vi "ReadWrite Top Level.vi"(5 "Late?":bool, 6 "Iteration":i32, 7 "Mode":T16, 8 "error in (no error)":errorcluster, 9 "Iteration Duration":i64, 11 "RT Data in":T1 {"Label Transfer Config"."Block Data Refs"."Data Reference" format="%.0x"; "Status Config"."HWOut Dur Ref" format="%.0x"; "Status Config"."HWIn Dur Ref" format="%.0x"; "Status Config"."HWOut Count Ref" format="%.0x"; "Status Config"."HWIn Count Ref" format="%.0x"; "Status Config"."Error Data Ref" format="%.0x"; "HWOutput Channels"."Labels Settings"."Driver Data"."Num Bits" min=1 max=32; "HWOutput Channels"."Labels Settings"."Driver Data"."Start Bit" min=8 max=31; "HWOutput Channels"."Labels Settings"."Block Data Refs"."Data Reference" format="%.0x"; "HWOutput Channels"."Labels Settings"."Label" format="%.0o"; "HWInput Channels"."Labels Settings"."Driver Data"."Num Bits" min=1 max=32; "HWInput Channels"."Labels Settings"."Driver Data"."Start Bit" min=8 max=31; "HWInput Channels"."Labels Settings"."Block Data Refs"."Data Reference" format="%.0x"; "HWInput Channels"."Labels Settings"."Label" format="%.0o"}) -> (0 "error out":errorcluster, 3 "RT Data out":T1 {"Label Transfer Config"."Block Data Refs"."Data Reference" format="%.0x"; "Status Config"."HWOut Dur Ref" format="%.0x"; "Status Config"."HWIn Dur Ref" format="%.0x"; "Status Config"."HWOut Count Ref" format="%.0x"; "Status Config"."HWIn Count Ref" format="%.0x"; "Status Config"."Error Data Ref" format="%.0x"; "HWOutput Channels"."Labels Settings"."Driver Data"."Num Bits" min=1 max=32; "HWOutput Channels"."Labels Settings"."Driver Data"."Start Bit" min=8 max=31; "HWOutput Channels"."Labels Settings"."Block Data Refs"."Data Reference" format="%.0x"; "HWOutput Channels"."Labels Settings"."Label" format="%.0o"; "HWInput Channels"."Labels Settings"."Driver Data"."Num Bits" min=1 max=32; "HWInput Channels"."Labels Settings"."Driver Data"."Start Bit" min=8 max=31; "HWInput Channels"."Labels Settings"."Block Data Refs"."Data Reference" format="%.0x"; "HWInput Channels"."Labels Settings"."Label" format="%.0o"})   [LabVIEW 2011, in "AIT 1553 Custom Device.lvlib"]
uses:
  AIT 1553 Custom Device.lvlib
  RT Controls/ReadWrite Selector.ctl
  RT Controls/RT Data.ctl
  RT Controls/RT HW Channel.ctl
  RT Controls/RT Label Settings.ctl
  Controls and Global/Label.ctl
  Controls and Global/transferPeriod.ctl
  <vilib>/NI Veristand/Custom Device API/Block Data Reference.ctl
  <vilib>/NI Veristand/Custom Device API/Data Reference.ctl
  RT Controls/Driver Data.ctl
  Controls and Global/Start Bit.ctl
  Controls and Global/Number of Bits.ctl
  RT Controls/Error Qs.ctl
  RT Controls/Status Channels Config.ctl
  RT Controls/FIFO.ctl
  RT Controls/Label Transfer Config.ctl
  <userlib>/ARINC-429/vi/enum/Owl429HardwareSource.ctl
  <vilib>/NI Veristand/Custom Device API/NI VeriStand - Set Channel Value by Data Reference.vi
  <vilib>/NI Veristand/Custom Device API/NI VeriStand - Get Channel Values by Block Data Reference.vi
  <vilib>/NI Veristand/Custom Device API/Global Data Refs.vi
  <vilib>/NI Veristand/Custom Device API/Custom Device API.lvlib
  <userlib>/ARINC-429/Owl429.lvlib
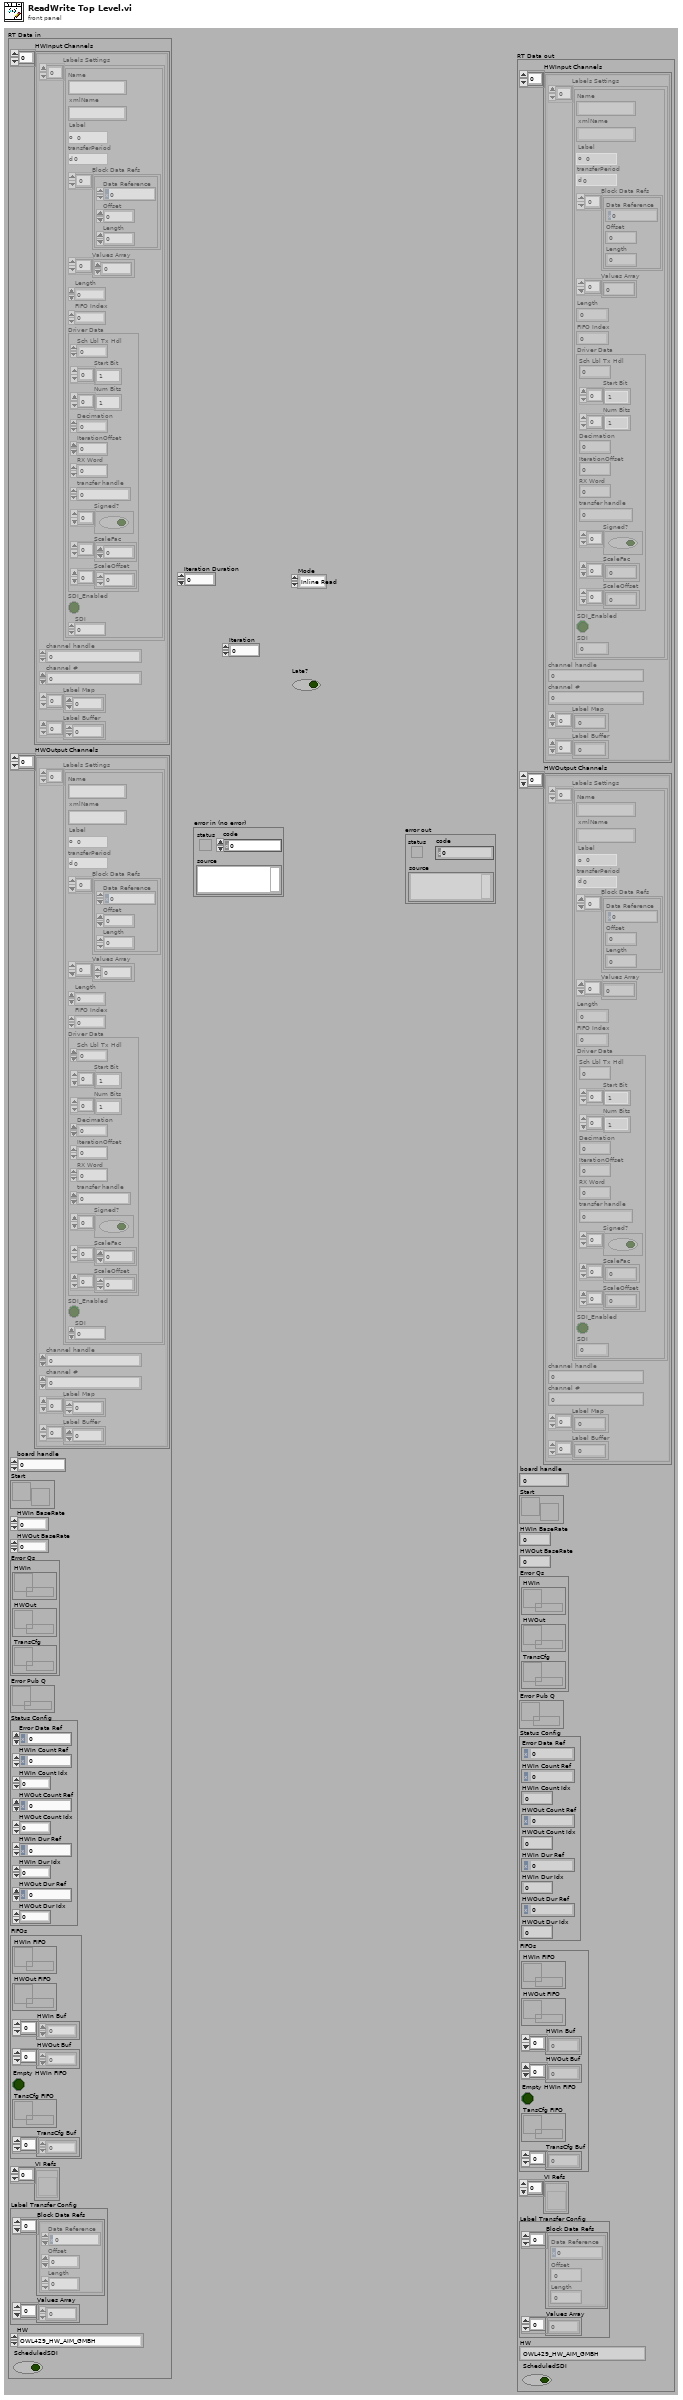
[diagram p1: front panel]
types:
  T1 = typedef "AIT 1553 Custom Device.lvlib/RT Data.ctl" = cluster{"HWInput Channels":T2[], "HWOutput Channels":T2[], "board handle":u32, "Start":refnum<notifier>, "HWIn BaseRate":i64, "HWOut BaseRate":i64, "Error Qs":T11, "Error Pub Q":refnum<queue>, "Status Config":T12, "FIFOs":T13, "VI Refs":refnum<vi>[], "Label Transfer Config":T14, "HW":T15, "ScheduledSDI":bool}
  T2 = typedef "AIT 1553 Custom Device.lvlib/RT HW Channel.ctl" = cluster{"Labels Settings":T3[], "channel handle":u32, "channel #":u16, "Label Map":i32[], "Label Buffer":u32[]}
  T3 = typedef "AIT 1553 Custom Device.lvlib/RT Label Settings.ctl" = cluster{"Name":string, "xmlName":string, "Label":T4, "transferPeriod":T5, "Block Data Refs":T6[], "Values Array":dbl[], "Length":i32, "FIFO Index":i32, "Driver Data":T8, "SDI_Enabled":bool, "SDI":u8}
  T4 = typedef "AIT 1553 Custom Device.lvlib/Label.ctl" = u8
  T5 = typedef "AIT 1553 Custom Device.lvlib/transferPeriod.ctl" = u32
  T6 = typedef "Custom Device API.lvlib/Block Data Reference.ctl" = cluster{"Data Reference":T7, "Offset":i32, "Length":i32}
  T7 = typedef "Custom Device API.lvlib/Data Reference.ctl" = i32
  T8 = typedef "AIT 1553 Custom Device.lvlib/Driver Data.ctl" = cluster{"Sch Lbl Tx Hdl":u32, "Start Bit":T9[], "Num Bits":T10[], "Decimation":i32, "IterationOffset":i32, "RX Word":u32, "transfer handle":u32, "Signed?":bool[], "ScaleFac":dbl[], "ScaleOffset":dbl[]}
  T9 = typedef "AIT 1553 Custom Device.lvlib/Start Bit.ctl" = i32
  T10 = typedef "AIT 1553 Custom Device.lvlib/Number of Bits.ctl" = i32
  T11 = typedef "AIT 1553 Custom Device.lvlib/Error Qs.ctl" = cluster{"HWIn":refnum<queue>, "HWOut":refnum<queue>, "TransCfg":refnum<queue>}
  T12 = typedef "AIT 1553 Custom Device.lvlib/Status Channels Config.ctl" = cluster{"Error Data Ref":T7, "HWIn Count Ref":T7, "HWIn Count Idx":i32, "HWOut Count Ref":T7, "HWOut Count Idx":i32, "HWIn Dur Ref":T7, "HWIn Dur Idx":i32, "HWOut Dur Ref":T7, "HWOut Dur Idx":i32}
  T13 = typedef "AIT 1553 Custom Device.lvlib/FIFO.ctl" = cluster{"HWIn FIFO":refnum<k33>, "HWOut FIFO":refnum<k33>, "HWIn Buf":dbl[], "HWOut Buf":dbl[], "Empty HWIn FIFO":bool, "TansCfg FIFO":refnum<k33>, "TransCfg Buf":dbl[]}
  T14 = typedef "AIT 1553 Custom Device.lvlib/Label Transfer Config.ctl" = cluster{"Block Data Refs":T6[], "Values Array":dbl[]}
  T15 = typedef "Owl429.lvlib/Owl429HardwareSource.ctl" = enum16{"OWL429_HW_AIM_GMBH", "OWL429_HW_AIT"}
  T16 = typedef "AIT 1553 Custom Device.lvlib/ReadWrite Selector.ctl" = enum16{"Inline Read", "Inline Write", "Async HWIn", "Async HWOut"}
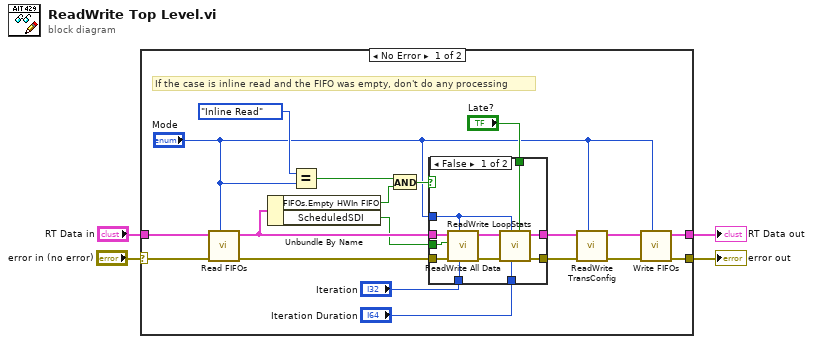
[diagram p0: block diagram]
diagram:
  n1 = case shown="No Error" "error in (no error)" {
    selector: "error in (no error)" -> [w13 w38]
    tunnel: "RT Data in" -> [w23 w37]
    tunnel: [w22 w37] -> w3
    tunnel: [w21 w38] -> w2
    frame No Error {
      # "If the case is inline read and the FIFO was empty, don't do any processing"
      n2 = call "Read FIFOs.vi"("Mode"="Mode", "error in (no error)"=w13, "RT Data in"=w23) -> ("error out"=w20:errorcluster, "RT Data out"=w17:T1)  [unwired: 7 in]
      n3 = Unbundle By Name(w17) -> ("FIFOs.Empty HWIn FIFO"=w16:bool, "ScheduledSDI"=w5:bool)
      n4 = Equal?(x=ReadWrite_Selector."Inline Read", y="Mode") -> (x = y?=w18:bool)
      n5 = And(x=w18, y=w16) -> (x .and. y?=w15:bool)
      n6 = case shown="False" w15 {
        tunnel: w20 -> [w34 w36]
        tunnel: [w29 w36] -> w10
        tunnel: [w28 w35] -> w9
        tunnel: w17 -> [w33 w35]
        tunnel: "Mode" -> [w26 _]
        tunnel: "Iteration" -> [w32 _]
        tunnel: "Late?" -> [w27 _]
        tunnel: "Iteration Duration" -> [w25 _]
        tunnel: w5 -> [w24 _]
        frame False {
          n7 = call "ReadWrite All Data.vi"("Iteration"=w32, "Mode"=w26, "error in (no error)"=w34, "ScheduledSDI"=w24, "RT Data in"=w33) -> ("error out"=w30:errorcluster, "RT Data out"=w31:T1)  [unwired: 5 in]
          n8 = call "ReadWrite LoopStats.vi"("Late"=w27, "Iteration Duration"=w25, "Mode"=w26, "error in (no error)"=w30, "RT Data in"=w31) -> ("error out"=w29:errorcluster, "RT Data out"=w28:T1)  [unwired: 5 in]
        }
        frame True {
        }
      }
      n9 = call "ReadWrite TransConfig.vi"("Mode"="Mode", "error in (no error)"=w10, "RT Data in"=w9) -> ("error out"=w6:errorcluster, "RT Data out"=w7:T1)  [unwired: 7 in]
      n10 = call "Write FIFOs.vi"("Mode"="Mode", "error in (no error)"=w6, "RT Data in"=w7) -> ("error out"=w21:errorcluster, "RT Data out"=w22:T1)  [unwired: 7 in]
    }
    frame Error {
    }
  }
  "error out" <- w2
  "RT Data out" <- w3
